vi "getCONNECTPayload.vi"(11 "CONNECT in":refnum<class "CONNECT.lvclass">) -> (2 "Payload":T1, 3 "CONNECT out":refnum<class "CONNECT.lvclass">)   [LabVIEW 2013, in "MQTT_Control_Packets.lvlib" / "CONNECT.lvclass"]
uses:
  CONNECT.lvclass
  ConnectPayload -- cluster.ctl
  ControlPacket/ControlPacket.lvclass/ControlPacket.ctl
  ControlPacket/ControlPacket.lvclass
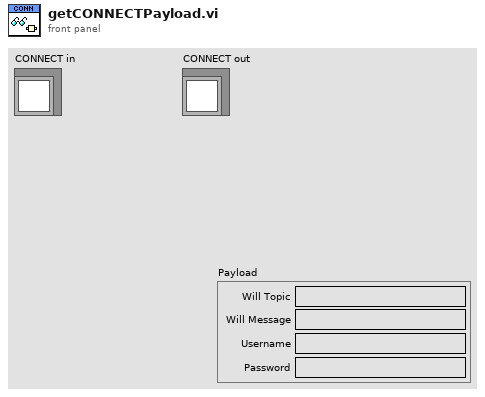
[diagram p1: front panel]
types:
  T1 = typedef "MQTT_Control_Packets.lvlib/CONNECT.lvclass/ConnectPayload -- cluster.ctl" = cluster{"Will Topic":string, "Will Message":string, "Username":string, "Password":string}
  T2 = typedef "MQTT_Control_Packets.lvlib/CONNECT.lvclass/ConnectFlags -- cluster.ctl" = cluster{"Reserved":bool, "Clean Session":bool, "Will Flag":bool, "Will QoS 1":bool, "Will QoS 2":bool, "Will Retain":bool, "Password Flag":bool, "User Name Flag":bool}
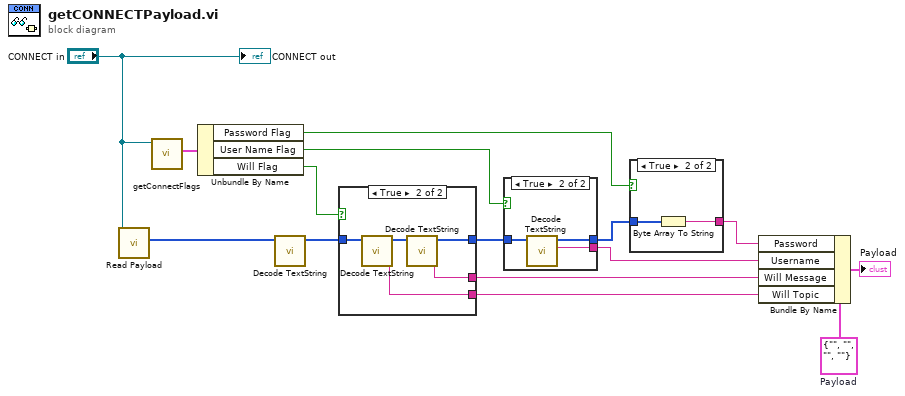
[diagram p0: block diagram]
diagram:
  w13 = T1 {"Will Topic"="", "Will Message"="", "Username"="", "Password"=""}  # Payload
  n1 = call "Read Payload.vi"("ControlPacket in"="CONNECT in") -> ("Payload"=w11:u8[])  [unwired: 9 in, 1 out]
  n2 = call "getConnectFlags.vi"("CONNECT in"="CONNECT in") -> ("Connect Flags"=w14:T2)  [unwired: 9 in, 1 out]
  n3 = Unbundle By Name(w14) -> ("Password Flag"=w1:bool, "User Name Flag"=w5:bool, "Will Flag"=w10:bool)
  n4 = call "Decode TextString.vi"("Length-Prefixed Field"=w11) -> ("Remaining Packets"=w9:u8[])  [unwired: 8 in, 2 out]
  n5 = case shown="True" w10 {
    tunnel: w9 -> [w16 w21]
    tunnel: [w16 w19] -> w6
    tunnel: [_ w18] -> w8
    tunnel: [_ w17] -> w7
    frame False {
    }
    frame True {
      n6 = call "Decode TextString.vi"("Length-Prefixed Field"=w21) -> ("Text String"=w18:string, "Remaining Packets"=w20:u8[])  [unwired: 8 in, 1 out]
      n7 = call "Decode TextString.vi"("Length-Prefixed Field"=w20) -> ("Text String"=w17:string, "Remaining Packets"=w19:u8[])  [unwired: 8 in, 1 out]
    }
  }
  n8 = case shown="True" w5 {
    tunnel: w6 -> [w22 w25]
    tunnel: [w22 w24] -> w3
    tunnel: [_ w23] -> w4
    frame False {
    }
    frame True {
      n9 = call "Decode TextString.vi"("Length-Prefixed Field"=w25) -> ("Text String"=w23:string, "Remaining Packets"=w24:u8[])  [unwired: 8 in, 1 out]
    }
  }
  n10 = case shown="True" w1 {
    tunnel: w3 -> [_ w27]
    tunnel: [_ w26] -> w2
    frame False {
    }
    frame True {
      n11 = Byte Array To String(unsigned byte array=w27) -> (string=w26:string)
    }
  }
  n12 = Bundle By Name(cluster=w13, "Password"=w2, "Username"=w4, "Will Message"=w7, "Will Topic"=w8) -> (→"Payload":T1)
  "CONNECT out" <- "CONNECT in"
